vi "Simple Math.vi"() -> ()   [LabVIEW 2010]
panel:
  out "Round LED":bool
  out "AxB":dbl
  out "A+B":dbl
  in  "B":dbl
  in  "A":dbl
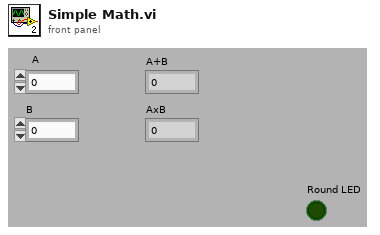
[diagram p1: front panel]
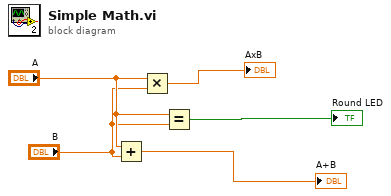
[diagram p0: block diagram]
diagram:
  n1 = Add(x="A", y="B") -> (x+y=→"A+B":dbl)
  n2 = Multiply(x="A", y="B") -> (x*y=→"AxB":dbl)
  n3 = Equal?(x="A", y="B") -> (x = y?=→"Round LED":bool)
